vi "SubVI_Stuetzpunkte.vi"(8 "error in (no error)":errorcluster, 9 "y-Wert":dbl[](array[numeric]), 10 "x-Wert":dbl[](array[numeric]), 11 "x-Value":dbl) -> (0 "error out":errorcluster, 1 "Numeric":dbl, 2 "Numeric 3":dbl, 3 "Index":i32=2, 4 "Numeric 4":dbl, 5 "Numeric 2":dbl)   [LabVIEW 2020]
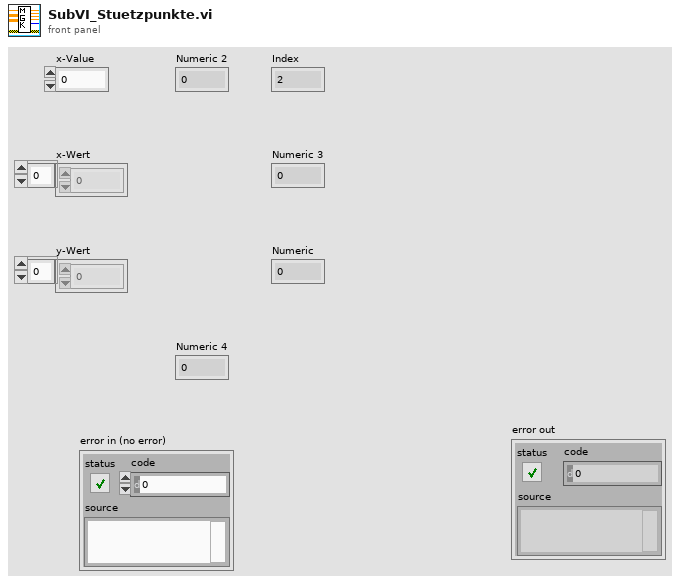
[diagram p1: front panel]
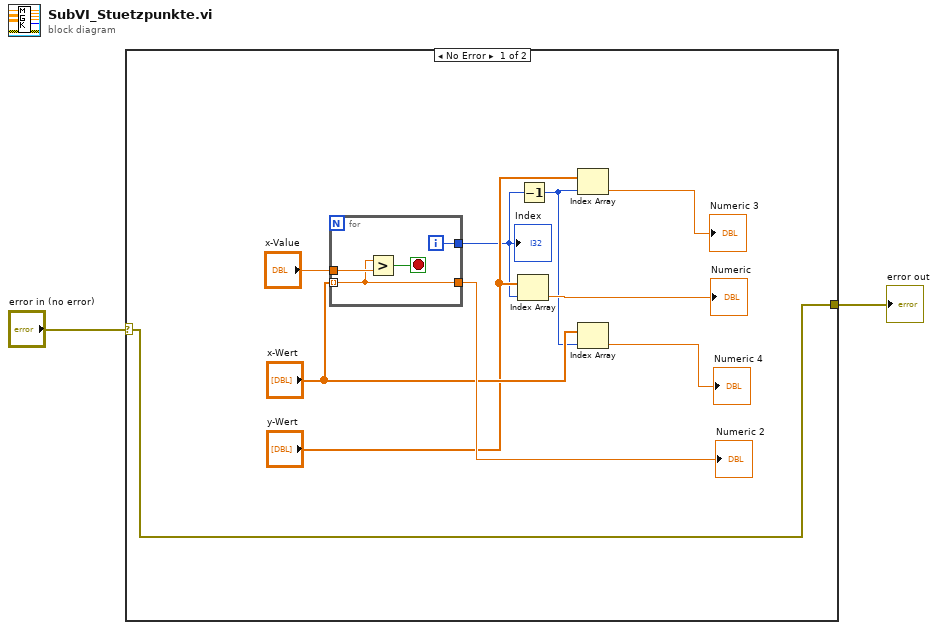
[diagram p0: block diagram]
diagram:
  n1 = case shown="No Error" "error in (no error)" {
    selector: "error in (no error)" -> [w3 w17]
    tunnel: [w3 w17] -> w1
    frame No Error {
      n2 = for {
        tunnel: "x-Wert" -> [w14] mode=indexing
        tunnel: "x-Value" -> [w16]
        tunnel: [w14] -> w11
        tunnel: [w13] -> w4
        i -> [w13]
        stop <- w15 stop-if-true
        n3 = Greater?(x=w14, y=w16) -> (0:w15:bool)
      }
      "Index" <- w4
      "Numeric 2" <- w11
      n4 = Index Array(array="y-Wert", index=w4) -> (element=→"Numeric":dbl)
      n5 = Decrement(x=w4) -> (x-1=w5:i32)
      n6 = Index Array(array="y-Wert", index=w5) -> (element=→"Numeric 3":dbl)
      n7 = Index Array(array="x-Wert", index=w5) -> (element=→"Numeric 4":dbl)
    }
    frame Error {
    }
  }
  "error out" <- w1
